vi "Simple AAP.vi"() -> ()   [LabVIEW 2014]
panel:
  out "Average Value":dbl
  out "Waveform Graph":dynamicdata(graph)
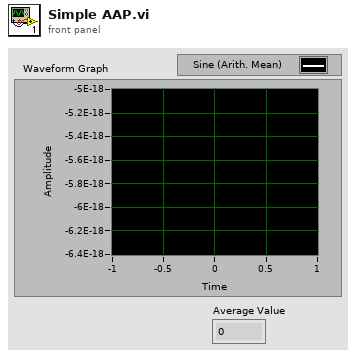
[diagram p1: front panel]
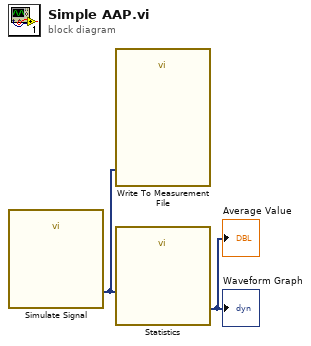
[diagram p0: block diagram]
diagram:
  n1 = call "Simulate Signal"() -> ("Sine"=w1:dynamicdata)  [unwired: 14 in, 1 out]
  n2 = call "Write To Measurement File"("Signals"=w1) -> ()  [unwired: 16 in, 3 out]
  n3 = call "Statistics"("Signals"=w1) -> ("Arithmetic Mean"=→"Waveform Graph" →"Average Value":dynamicdata)  [unwired: 25 in, 1 out]
